vi "Get Automatic Execution On Power On.vi"(4 "error in (no error)":errorcluster, 7 "VISA resource name":refnum<visa-resource-name>) -> (0 "error out":errorcluster, 1 "Number of times of execution":i32=1, 2 "Program Number":i32=1, 3 "VISA resource name out":refnum<visa-resource-name>)   [LabVIEW 2012, in "Newport ESP301.lvlib"]
doc: "reports the number of the program that is executed on power on and the number of times of execution."
uses:
  Newport ESP301.lvlib
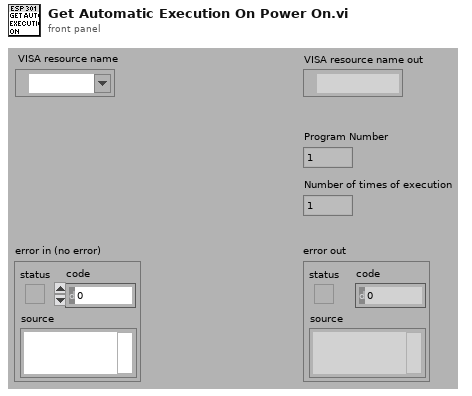
[diagram p1: front panel]
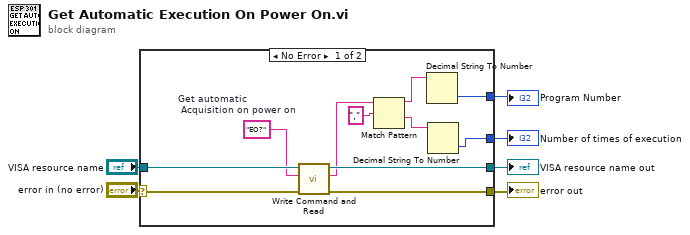
[diagram p0: block diagram]
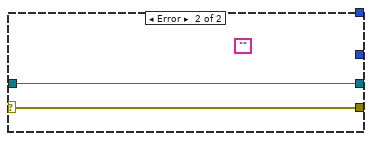
[diagram p2: hidden frame]
diagram:
  n1 = case shown="No Error" "error in (no error)" {
    selector: "error in (no error)" -> [w15 w19]
    tunnel: [w13 w19] -> w6
    tunnel: "VISA resource name" -> [w17 w18]
    tunnel: [w16 w18] -> w5
    tunnel: [w9 _] -> w2
    tunnel: [w8 _] -> w1
    frame No Error {
      w14 = "EO?"  # Get automatic  Acquisition on power on
      n2 = call "Write Command and Read.vi"("error in (no error)"=w15, "Command"=w14, "VISA resource name"=w17) -> ("error out"=w13:errorcluster, "Returned string"=w7:string, "VISA resource name out"=w16:refnum<visa-resource-name>)  [unwired: 4 in]
      n3 = Match Pattern(string=w7, regular expression="," ("expression régulière")) -> (before substring=w11:string, after substring=w10:string)  [unwired: 1 in, 2 out]
      n4 = Decimal String To Number(string=w11) -> (number=w8:i32)  [unwired: 2 in, 1 out]
      n5 = Decimal String To Number(string=w10) -> (number=w9:i32)  [unwired: 2 in, 1 out]
    }
    frame Error {
      (unwired) ""
    }
  }
  "error out" <- w6
  "VISA resource name out" <- w5
  "Program Number" <- w1
  "Number of times of execution" <- w2
